vi "About APP generic.vi"() -> ()   [LabVIEW 2013]
panel:
  in  "About":bool
  in  "OK":bool
  # "APPLICATION NAME"
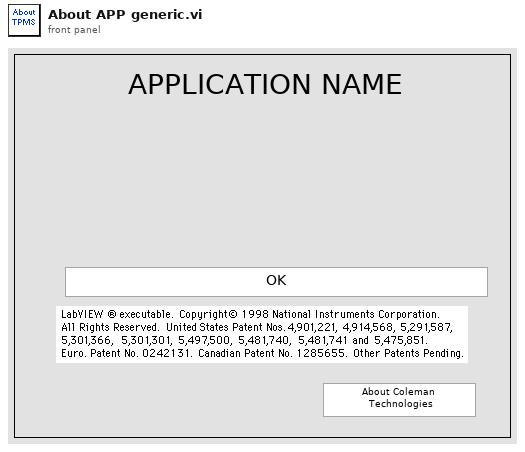
[diagram p1: front panel]
types:
  T1 = cluster{"left":i16, "top":i16, "right":i16, "bottom":i16}
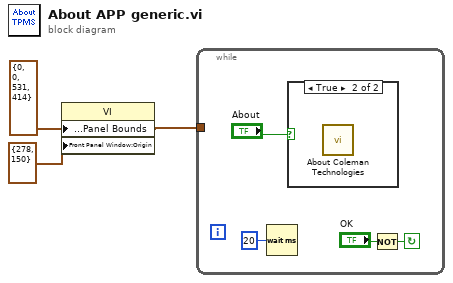
[diagram p0: block diagram]
diagram:
  w1 = T1 {"left"=0, "top"=0, "right"=531, "bottom"=414} ("Front Panel Window:Panel Bounds")
  n1 = property class="VI"("Front Panel Window:Panel Bounds"=w1, "Front Panel Window:Origin"=cluster{"Horizontal":i16, "Vertical":i16} {"Horizontal"=278, "Vertical"=150}) -> ()  [unwired: 2 in, 2 out]
  n2 = while {
    tunnel: w1 -> [_]
    stop <- w6 continue-if-true
    n3 = Wait (ms)(milliseconds to wait=u32 20) -> ()  [unwired: 1 out]
    n4 = case shown="True" "About" {
      frame False {
      }
      frame True {
        n5 = call "About Coleman Technologies.vi"() -> ()  [unwired: 1 out]
      }
    }
    n6 = Not(x="OK") -> (.not. x?=w6:bool)
  }
